vi "Pulsecounter.vi"() -> ()   [LabVIEW 2011]
panel:
  in  "PulseCounter":i32
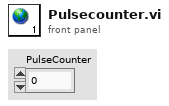
[diagram p1: front panel]
diagram:
